vi "Write Shutters to Initialize.vi"(8 "error in (no error)":errorcluster, 10 "Shutters to Initialize":T1[](array[typedef]), 11 "Uniblitz Shutter in":refnum<class "Uniblitz Shutter.lvclass">) -> (0 "error out":errorcluster, 3 "Uniblitz Shutter out":refnum<class "Uniblitz Shutter.lvclass">)   [LabVIEW 2015, in "Uniblitz Shutter.lvlib" / "Uniblitz Shutter.lvclass"]
uses:
  Uniblitz Shutter.lvclass
  Resources/Type Defs/Excitation.ctl
  Resources/Type Defs/Shutter Configuration.ctl
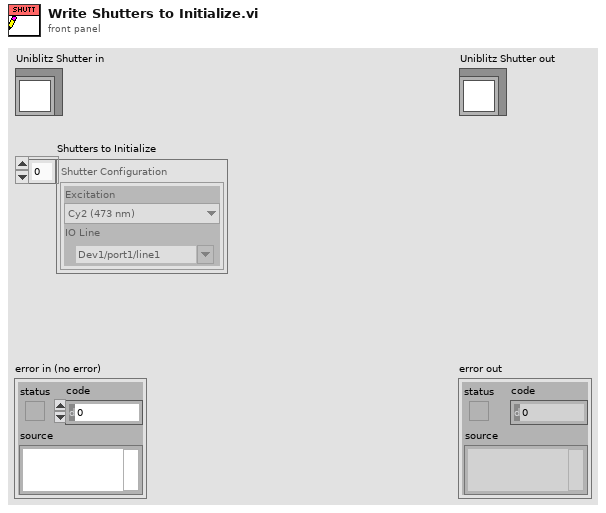
[diagram p1: front panel]
types:
  T1 = typedef "Shutter Configuration.ctl" = cluster{"Excitation":T2, "IO Line":tag}
  T2 = typedef "Excitation.ctl" = enum16{"Cy2 (473 nm)", "Cy3 (532 nm)", "Cy5 (639 nm)", "Cy7 (730 nm)"}
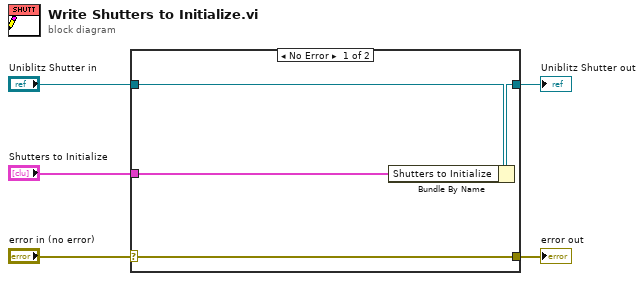
[diagram p0: block diagram]
diagram:
  n1 = case shown="No Error" "error in (no error)" {
    selector: "error in (no error)" -> [w9 w10]
    tunnel: [w9 w10] -> w4
    tunnel: [w7 w11] -> w2
    tunnel: "Uniblitz Shutter in" -> [w8 w11]
    tunnel: "Shutters to Initialize" -> [w6 _]
    frame No Error {
      n2 = Bundle By Name(cluster=w8, "Shutters to Initialize"=w6) -> (w7:refnum<class "Uniblitz Shutter.lvclass">)
    }
    frame Error {
    }
  }
  "error out" <- w4
  "Uniblitz Shutter out" <- w2
